vi "未命名 1.vi"() -> ()   [LabVIEW 2020]
uses:
  <instrlib>/Keithley 27XX/Public/Data/Read Multiple Direct.vi
  <instrlib>/Keithley 27XX/Keithley 27XX.lvlib
panel:
  out "error out":errorcluster
  out "Measurement Data":dbl[](array[numeric])
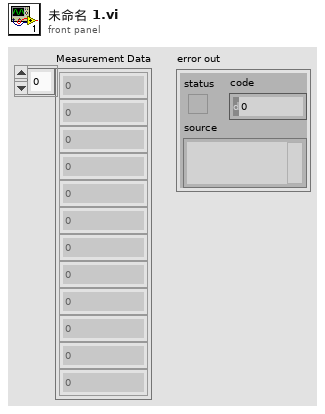
[diagram p1: front panel]
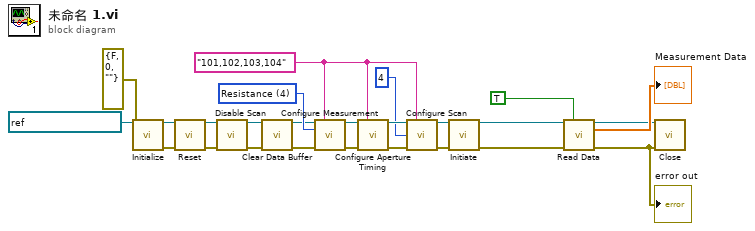
[diagram p0: block diagram]
diagram:
  w15 = u16 4 items=["DC Voltage", "AC Voltage", "DC Current", "AC Current", "Resistance", "Four-Wire Resistance", "Temperature", "Frequency", "Period", "Continuity"] ("Function (0: DC Voltage)")
  w12 = "101,102,103,104" ("Scan List (Empty)")
  n1 = call <instrlib>:"Initialize.vi"("VISA resource name"=refnum<visa-resource-name> "Keithley2700-1", "error in (no error)"=errorcluster {"status"=FALSE, "code"=0, "source"=""}) -> ("VISA resource name out"=w25:refnum<visa-resource-name>, "error out"=w13:errorcluster)  [unwired: 12 in]
  n2 = call <instrlib>:"Reset.vi"("VISA resource name"=w25, "error in (no error)"=w13) -> ("VISA resource name out"=w11:refnum<visa-resource-name>, "error out"=w10:errorcluster)  [unwired: 12 in]
  n3 = call <instrlib>:"Disable Scan.vi"("VISA resource name"=w11, "error in (no error)"=w10) -> ("VISA resource name out"=w4:refnum<visa-resource-name>, "error out"=w5:errorcluster)  [unwired: 12 in]
  n4 = call <instrlib>:"Clear Data Buffer.vi"("VISA resource name"=w4, "error in (no error)"=w5) -> ("VISA resource name out"=w3:refnum<visa-resource-name>, "error out"=w2:errorcluster)  [unwired: 12 in]
  n5 = call <instrlib>:"Configure Measurement.vi"("VISA resource name"=w3, "Scan List (Empty)"=w12, "Function (0: DC Voltage)"=w15, "error in (no error)"=w2) -> ("VISA resource name out"=w21:refnum<visa-resource-name>, "error out"=w24:errorcluster)  [unwired: 10 in]
  n6 = call <instrlib>:"Configure Aperture Timing.vi"("VISA resource name"=w21, "Scan List (Empty)"=w12, "error in (no error)"=w24) -> ("VISA resource name out"=w22:refnum<visa-resource-name>, "error out"=w23:errorcluster)  [unwired: 11 in]
  n7 = call <instrlib>:"Configure Scan.vi"("VISA resource name"=w22, "Channel List (101:110)"=w12, "Sample Count (100)"=4, "error in (no error)"=w23) -> ("VISA resource name out"=w7:refnum<visa-resource-name>, "error out"=w9:errorcluster)  [unwired: 10 in]
  n8 = call <instrlib>:"Initiate.vi"("VISA resource name"=w7, "error in (no error)"=w9) -> ("VISA resource name out"=w6:refnum<visa-resource-name>, "error out"=w8:errorcluster)  [unwired: 12 in]
  n9 = call-poly <instrlib>:"Read Data.vi"("VISA resource name"=w6, "All Data Elements (False)"=TRUE, "error in (no error)"=w8) -> ("VISA resource name out"=w17:refnum<visa-resource-name>, "Measurement Data"=→"Measurement Data":dbl[], "error out"=w16:errorcluster)  [unwired: 7 in, 3 out]
  "error out" <- w16
  n10 = call <instrlib>:"Close.vi"("VISA resource name"=w17, "error in (no error)"=w16) -> ()  [unwired: 13 in, 1 out]
